vi "GUI_Frontend.vi"() -> ()   [LabVIEW 2013]
uses:
  Shared/GUI_Template/GUI_master/tcp new data cluster.ctl
  Shared/GUI_Template/GUI_master/tcp_new_data_event.ctl
panel:
  in  "Refresh Button":bool
  out "Amp0 Energy Out":dbl(graph)=0.002414
  in  "GUIdevice 3":string="DS-LaserFrontEndLogger"
  in  "reading.var 6::3":dbl=0.002385 caption="Amp0 pulse energy" min=-100000.0 max=100000.0
  in  "Position.Axis 132::2":dbl=7270.0 caption="Pos. Motor Axis 2" min=-999999.0 max=999999.0 format="%#_6f"
  in  "Position.Axis 131::2":dbl=8590.0 caption="Pos. Motor Axis 1" min=-999999.0 max=999999.0 format="%#_6f"
  in  "GUIdevice 2":string="Picopad23"
  in  "Target.Y::1":dbl=467.0 caption="T1y" min=1.0 max=600.0 format="%#_6f"
  in  "Target.X::1":dbl=369.0 caption="T1x" min=1.0 max=800.0 format="%#_6f"
  in  "stop":bool
  out "image::1":T1(plugin-control) caption="XPW Output"
  in  "GUIdevice 1":string="XPW_cam"
  out "tcp data event":T2
  out "error IO 2":errorcluster
  # "Pico Control"
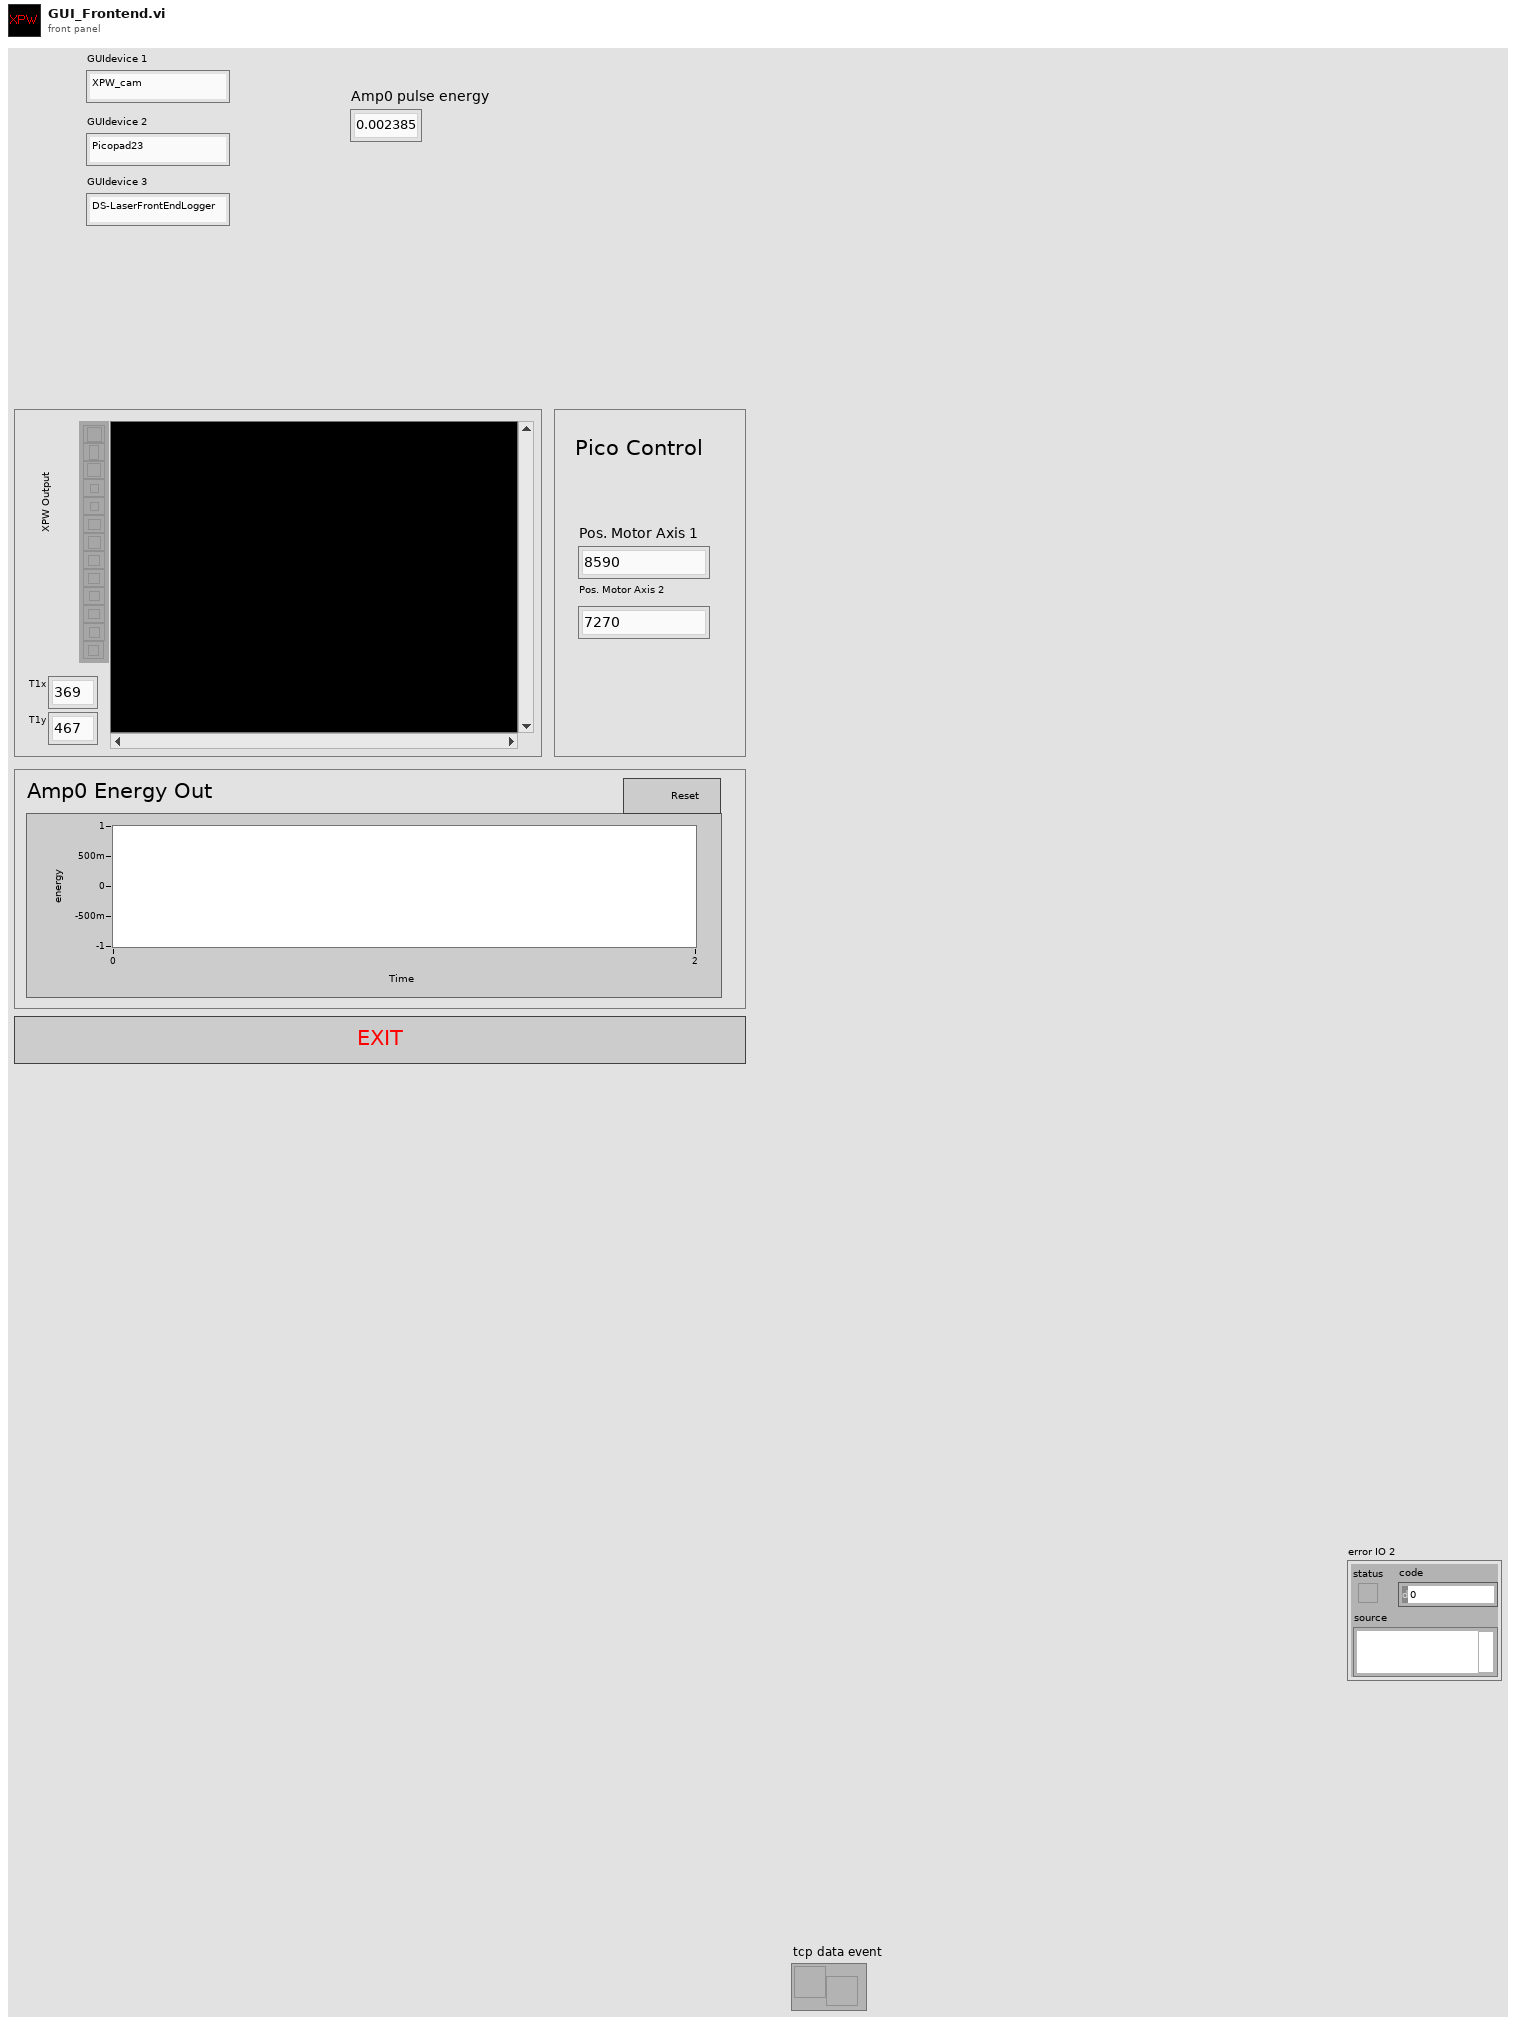
[diagram p1: front panel]
types:
  T1 = typedef "IMAQ Image.ctl" = refnum<image>
  T2 = typedef "tcp_new_data_event.ctl" = refnum<user-event>
  T3 = typedef "tcp new data cluster.ctl" = cluster{"EventEnum":enum16{"new data", "connection status update"}, "Device name":string}
  T4 = cluster{"Left":i32, "Top":i32, "Right":i32, "Bottom":i32}
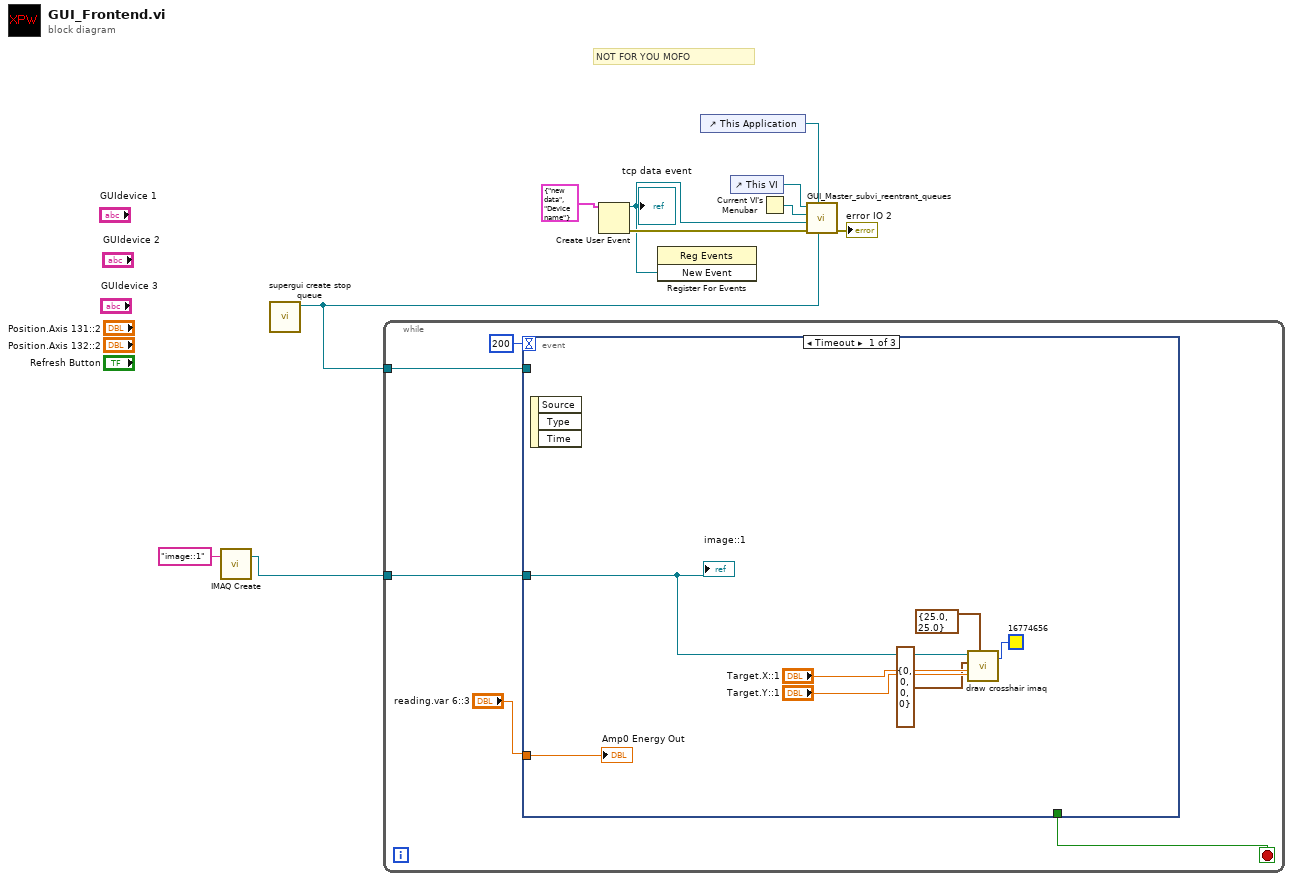
[diagram p0: block diagram]
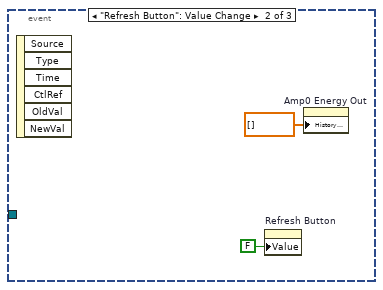
[diagram p2: hidden frame]
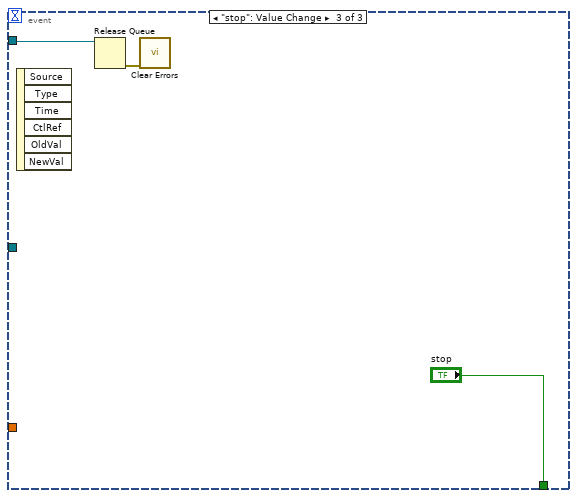
[diagram p3: hidden frame]
diagram:
  # "NOT FOR YOU MOFO"
  n1 = call "IMAQ Create"("Image Name"="image::1") -> ("New Image"=w2:T1)  [unwired: 4 in, 1 out]
  n2 = call "supergui create stop queue.vi"() -> ("STOP Queue out"=w1:refnum<queue>)  [unwired: 11 in]
  n3 = while {
    tunnel: w2 -> [w13]
    tunnel: w1 -> [w11]
    stop <- w15 stop-if-true
    n4 = event shown="[0] Timeout" {
      selector: _ -> [_ _ _]
      dyn-events: _ -> [_ _ _]
      timeout: 200 -> [_ _ _]
      tunnel: [_ _ "stop"] -> w15
      tunnel: w13 -> [w17 _ _]
      tunnel: "reading.var 6::3" -> [w16 _ _]
      tunnel: w11 -> [_ _ w26]
      event Timeout {
        n5 = event-data() -> ()  [unwired: 1 in, 3 out]
        n6 = call "draw crosshair imaq.vi"(5:u32 16774656 ("Color"), 6:"Target.Y::1", "clear overlay"=cluster{"xhair size":dbl, "xhair size 2":dbl} {"xhair size"=25.0, "xhair size 2"=25.0} ("size"), "Crosshair"="Target.X::1", "Bounding Rectangle"=T4 {"Left"=0, "Top"=0, "Right"=0, "Bottom"=0}, "image in"=w17) -> ()  [unwired: 4 in, 2 out]
        "image::1" <- w17
        "Amp0 Energy Out" <- w16
      }
      event "Refresh Button": Value Change {
        n7 = event-data() -> ()  [unwired: 1 in, 6 out]
        n8 = property on="Refresh Button" class="Bool (strict)"("Value"=FALSE ("Refresh Button")) -> ()  [unwired: 2 in, 2 out]
        n9 = property on="Amp0 Energy Out" class="WFChart (strict)"("History Data"=dbl[] []) -> ()  [unwired: 2 in, 2 out]
      }
      event "stop": Value Change {
        n10 = event-data() -> ()  [unwired: 1 in, 6 out]
        n11 = Release Queue(queue=w26) -> (error out=w25:errorcluster)  [unwired: 2 in, 2 out]
        n12 = call <vilib>:"Clear Errors.vi"("error in (no error)"=w25) -> ()  [unwired: 6 in, 1 out]
      }
    }
  }
  n13 = Create User Event(user event datatype=T3 {"EventEnum"=enum."new data", "Device name"="Device name"} ("New Event")) -> (user event=w5:refnum<user-event>, error out=w6:errorcluster)  [unwired: 1 in]
  "tcp data event" <- w5
  n14 = register-events(w5) -> ()  [unwired: 2 in, 2 out]
  n15 = control-ref of="This Application"() -> (w4:refnum<vi>)
  n16 = control-ref of="This VI"() -> (w9:refnum<vi>)
  n17 = Current VI's Menubar() -> (w8:refnum<k9>)
  n18 = call "GUI_Master_subvi_reentrant_queues.vi"("STOP Queue in"=w1, "This Application"=w4, "error in (no error)"=w6, "tcp data event"=w5, "Caller menu reference"=w8, "Caller VI ref"=w9) -> ("error out"=→"error IO 2":errorcluster)  [unwired: 5 in]
